vi "Shooter Ready Detection.vi"(8 "Right RPM":dbl, 9 "Left RPM":dbl, 10 "Right RPM Target":dbl, 11 "Left RPM Target":dbl) -> (3 "Shooter Ready?":bool)   [LabVIEW 2015]
uses:
  Robot Global Data.vi
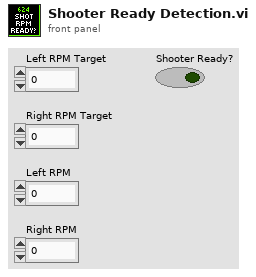
[diagram p1: front panel]
types:
  T1 = typedef "Dashboard Control Data.ctl" = cluster{"Auton Loops":dbl, "Shooter Presets":T2, "Encoder Control":T4, "Steer PID output":cluster{"output high":dbl, "output low":dbl}, " Steer PID gains":cluster{"proportional gain (Kc)":dbl, "integral time (Ti, min)":dbl, "derivative time (Td, min)":dbl}, "Drivetrain Settings":T5, "Vision Packet":T6, "Dashboard Drivetrain Command":T7}
  T2 = typedef "Shooter Presets.ctl" = cluster{"Batter Shot":T3, "Low Bar Curve Shot":T3, "Deep Middle Shot":T3, "Manual Shot":T3, "Left Ticks Per Rotation":dbl, "Right Ticks Per Rotation":dbl, "Low Bar Shot":T3, "Shooter RPM Tolerance":dbl, "IIR Filter Power":dbl}
  T3 = typedef "Shot Presets.ctl" = cluster{"Left Wheel RPM":dbl, "Right Wheel RPM":dbl}
  T4 = typedef "Encoder Control.ctl" = cluster{"Right Tick Constat":dbl, "Left Tick Constant":dbl, "Reset?":bool, "Y Dist":cluster{"PID gains":cluster{"proportional gain (Kc)":dbl, "integral time (Ti, min)":dbl, "derivative time (Td, min)":dbl}}, "Y Stop Thresh":dbl, "Y Stop Speed":dbl}
  T5 = typedef "Drivetrain Settings.ctl" = cluster{"Gyro Tolerance":dbl, "Throttle Ramp (ms)":dbl, "Angular rate compensation":bool, "Throttle to Rate Scale":dbl, "Rate compensation gain":dbl}
  T6 = typedef "Vision Packet.ctl" = cluster{"Distance":dbl, "Center X":dbl, "Center Y":dbl, "Found Target?":bool}
  T7 = typedef "Dashboard Drivetrain Command.ctl" = cluster{"Drivetrain Vision":T8, "Vision Scale Down Speed":dbl, "Vision PID gains":cluster{"proportional gain (Kc)":dbl, "integral time (Ti, min)":dbl, "derivative time (Td, min)":dbl}}
  T8 = typedef "Drivetrain Vision.ctl" = cluster{"High parameters":dbl, "Low parameters":dbl}
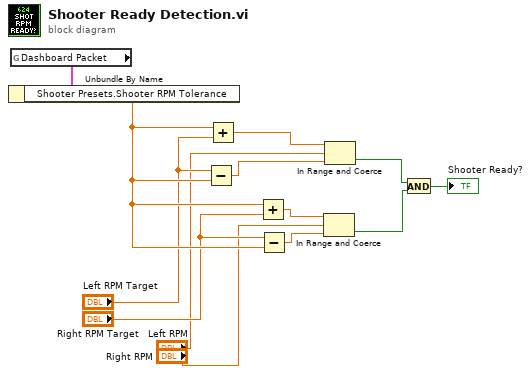
[diagram p0: block diagram]
diagram:
  n1 = global read "Robot Global Data.vi" "Dashboard Packet"() -> (w12:T1)
  n2 = Unbundle By Name(w12) -> ("Shooter Presets.Shooter RPM Tolerance"=w13:dbl)
  n3 = Subtract(x="Left RPM Target", y=w13) -> (x-y=w4:dbl)
  n4 = Add(x=w13, y="Left RPM Target") -> (x+y=w2:dbl)
  n5 = Add(x=w13, y="Right RPM Target") -> (x+y=w6:dbl)
  n6 = Subtract(x="Right RPM Target", y=w13) -> (x-y=w8:dbl)
  n7 = In Range and Coerce(upper limit=w6, x="Right RPM", lower limit=w8) -> (In Range?=w10:bool)  [unwired: 1 out]
  n8 = In Range and Coerce(upper limit=w2, x="Left RPM", lower limit=w4) -> (In Range?=w9:bool)  [unwired: 1 out]
  n9 = And(x=w9, y=w10) -> (x .and. y?=→"Shooter Ready?":bool)
